vi "06. Native MQTT Instrument.vi"(11 "QualifiedName":string="demo/system/instrument") -> ()   [LabVIEW 2019]
uses:
  Actor/Request -- cluster.ctl
  <vilib>/LabVIEW Open Source Project/MQTT Control Packets/Control Packets/ControlPacket/ControlPacket.lvclass/ControlPacket.ctl
  eb005712-7d9b-4db0-ad4b-d7048dbf5e76.vi
  d83398bf-d288-4447-9c56-1851baa950d7.vi
  3288b219-43a6-48ac-a265-cf9a9541cd0b.vi
  5f2e3dba-ef2d-4927-820c-bacd114549c6.vi
  <vilib>/JDP Science/JSONtext/Find Item.vi
  <vilib>/JDP Science/JSONtext/Next JSON Value.vi
  <vilib>/JDP Science/JSONtext/String Subset.vi
  <vilib>/JDP Science/JSONtext/Parsing/Advance past next JSON Value (inlined COPY).vi
  <vilib>/JDP Science/JSONtext/Parsing/Advance past whitespace.vi
  <vilib>/JDP Science/JSONtext/Parsing/Advance past String.vi
  <vilib>/JDP Science/JSONtext/Parsing/Advance past Number.vi
  <vilib>/JDP Science/JSONtext/Parsing/Advance past Line Ending.vi
  <vilib>/LabVIEW Open Source Project/MQTT Control Packets/Control Packets/PUBLISH/PUBLISH.lvclass
  C:/Program Files (x86)/National Instruments/LabVIEW 2019/vi.lib/LabVIEW Open Source Project/MQTT Control Packets/Control Packets/ControlPacket/ControlPacket.lvclass
  <vilib>/JDP Science/JSONtext/JSON text to Variant.vi
  <vilib>/Utility/error.llb/Error Cluster From Error Code.vi
  <vilib>/JDP Science/JSONtext/Parsing/Parse Full Path or Item Name.vi
  <vilib>/JDP Science/JSONtext/Parsing/Advance past Array.vi
  <vilib>/JDP Science/JSONtext/Parsing/Advance past Object.vi
  <vilib>/JDP Science/JSONtext/support/Error Cluster From Code.vi
  <vilib>/JDP Science/JSONtext/Offset/Find Item Locations by Path.vi
  <vilib>/JDP Science/JSONtext/LVClass Serializer/JSONtext LVClass Serializer.lvclass
  <vilib>/ErrorRing/Error Ring.xnode
  <vilib>/LabVIEW Open Source Project/MQTT Control Packets/Control Packets/ControlPacket/ControlPacket.lvclass
  <vilib>/JDP Science/JSONtext/JSONtext.lvlib
  <vilib>/ptbypt/NI_PtbyPt.lvlib
panel:
  in  "amplitude":dbl
  out "<JSON>Response":string
  out "<JSON>":string caption="<JSON>Request"
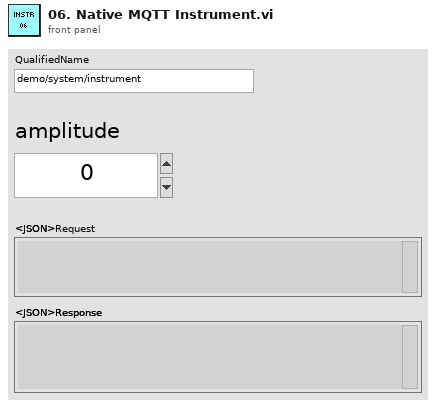
[diagram p1: front panel]
types:
  T1 = typedef "Actor Private Data.ctl" = cluster{"Client":refnum<class "Client.lvclass">, "QualifiedName":string, "EventReg":refnum<event-registration>, "Private Events":T2}
  T2 = typedef "Actor Private Events -- cluster.ctl" = cluster{"Stop":refnum<user-event>, "Subscribe":refnum<user-event>, "Unsubscribe":refnum<user-event>, "publish":refnum<user-event>}
  T3 = typedef "Request -- cluster.ctl" = cluster{"method":string, "<JSON>params":string, "id":string, "reply-topic":string}
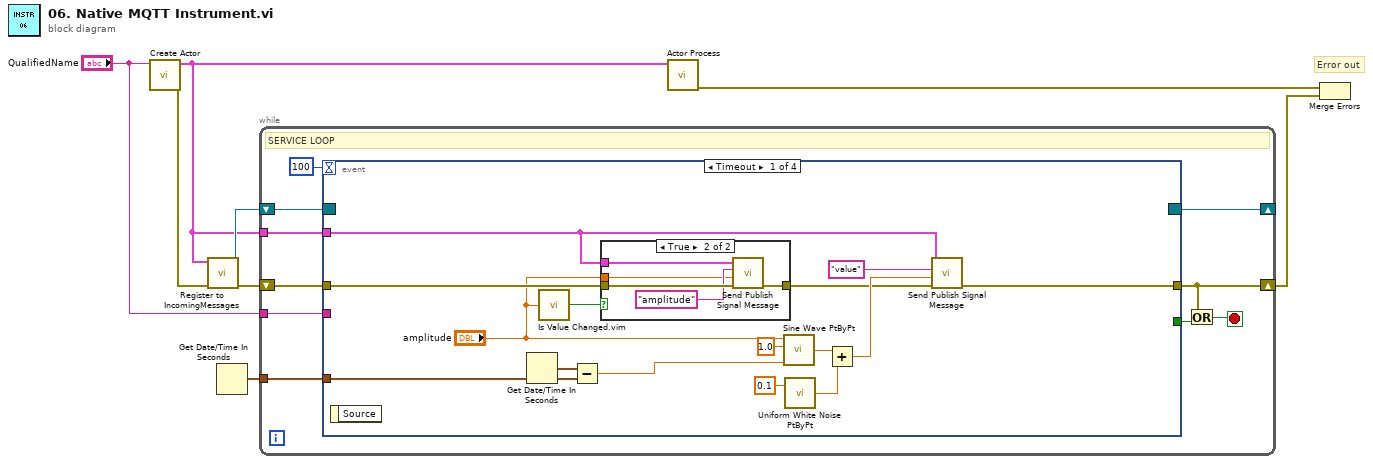
[diagram p0: block diagram]
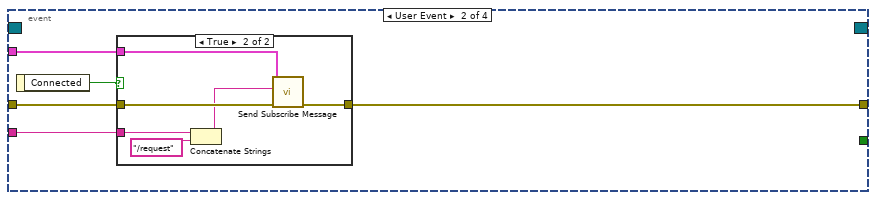
[diagram p3: hidden frame]
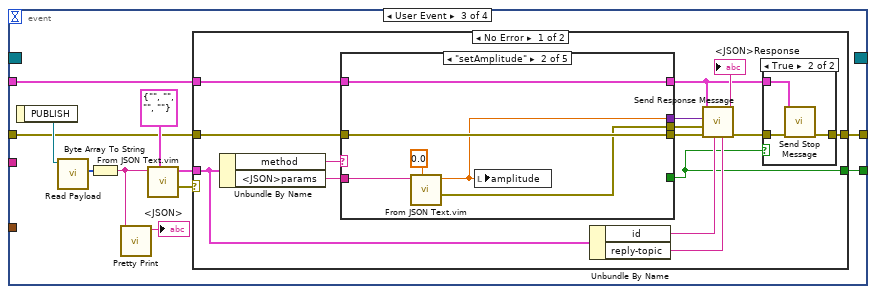
[diagram p5: hidden frame]
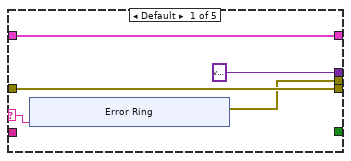
[diagram p7: hidden frame]
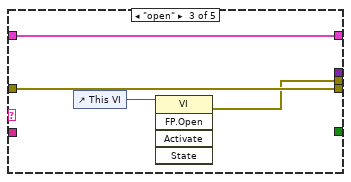
[diagram p8: hidden frame]
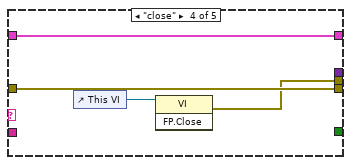
[diagram p9: hidden frame]
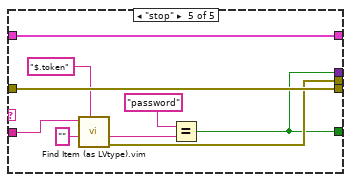
[diagram p10: hidden frame]
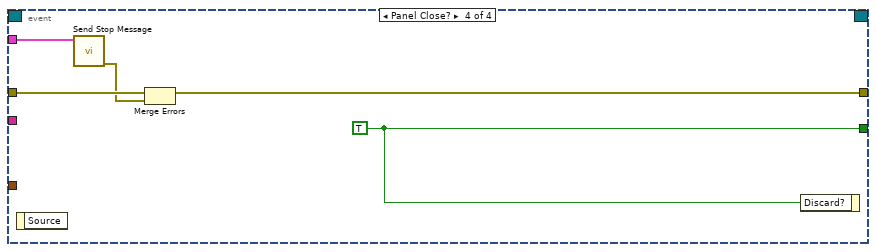
[diagram p12: hidden frame]
diagram:
  # "Error out"
  n1 = call "Create Actor.vi"("QualifiedName"="QualifiedName") -> ("error out"=w7:errorcluster, "Actor Class"=w5:T1)  [unwired: 9 in]
  n2 = call "Register to IncomingMessages.vi"("error in"=w7, "Actor Class"=w5) -> ("error out"=w4:errorcluster, "Incoming Messages"=w6:refnum<event-registration>)  [unwired: 8 in]
  n3 = Get Date/Time In Seconds() -> (seconds since 1Jan1904=w1:timestamp)
  n4 = while {
    tunnel: w5 -> [w16]
    shift-right: [w13] -> _
    shift-left: w6 -> [w14]
    shift-right: [w11] -> w3
    shift-left: w4 -> [w12]
    tunnel: "QualifiedName" -> [w10]
    tunnel: w1 -> [w9]
    stop <- w17 stop-if-true
    # "SERVICE LOOP"
    n5 = event shown="[0] Timeout" {
      selector: w14 -> [_ _ _ _]
      dyn-events: [_ _ _ _] -> w13
      timeout: 100 -> [_ _ _ _]
      tunnel: [_ _ w52 w122] -> w18
      tunnel: w16 -> [w24 w42 w57 w121]
      tunnel: [w28 w43 w55 w118] -> w11
      tunnel: w12 -> [w26 w44 w56 w120]
      tunnel: w10 -> [_ w40 _ _]
      tunnel: w9 -> [w20 _ _ _]
      event Timeout {
        n6 = event-data() -> ()  [unwired: 1 in, 1 out]
        n7 = Get Date/Time In Seconds() -> (seconds since 1Jan1904=w21:timestamp)
        n8 = call "Is Value Changed.vim"("value"="amplitude") -> ("changed or first call?"=w23:bool)
        n9 = Subtract(x=w21, y=w20) -> (x-y=w19:dbl)
        n10 = case shown="True" w23 {
          tunnel: w26 -> [w34 w39]
          tunnel: [w34 w38] -> w25
          tunnel: w24 -> [_ w36]
          tunnel: "amplitude" -> [_ w35]
          frame False {
          }
          frame True {
            n11 = call "Send Publish Signal Message.vi"("error in"=w39, "Variant"=w35, "Signal Name"="amplitude" ("Topic Name (empty: Payload name)"), "Actor Class"=w36) -> ("error out"=w38:errorcluster)  [unwired: 7 in]
          }
        }
        n12 = call <vilib>:"Sine Wave PtByPt.vi"("time"=w19, "frequency"=1.0, "amplitude"="amplitude") -> ("sine wave"=w33:dbl)  [unwired: 1 in]
        n13 = call <vilib>:"Uniform White Noise PtByPt.vi"("amplitude"=0.1) -> ("uniform white noise"=w31:dbl)  [unwired: 2 in]
        n14 = Add(x=w33, y=w31) -> (x+y=w29:dbl)
        n15 = call "Send Publish Signal Message.vi"("error in"=w25, "Variant"=w29, "Signal Name"="value" ("Topic Name (empty: Payload name)"), "Actor Class"=w24) -> ("error out"=w28:errorcluster)  [unwired: 7 in]
      }
      event User Event {
        n16 = event-data() -> ("Connected"=w41:bool)  [unwired: 1 in]
        n17 = case shown="True" w41 {
          tunnel: w44 -> [w45 w51]
          tunnel: [w45 w50] -> w43
          tunnel: w42 -> [_ w49]
          tunnel: w40 -> [_ w48]
          frame False {
          }
          frame True {
            n18 = Concatenate Strings(w48, "/request" ("QualifiedName")) -> (w46:string)
            n19 = call "Send Subscribe Message.vi"("error in"=w51, "Topic"=w46, "Actor Class"=w49) -> ("error out"=w50:errorcluster)  [unwired: 8 in]
          }
        }
      }
      event User Event {
        n20 = event-data() -> ("PUBLISH"=w62:refnum<class "PUBLISH.lvclass">)  [unwired: 1 in]
        n21 = call <vilib>:"Read Payload.vi"("ControlPacket in"=w62) -> ("Payload"=w61:u8[])  [unwired: 9 in, 1 out]
        n22 = Byte Array To String(unsigned byte array=w61) -> (string=w54:string)
        n23 = call <vilib>:"Pretty Print.vi"("JSON"=w54) -> ("<JSON>"=→"<JSON>":string)  [unwired: 8 in, 2 out]
        n24 = call "From JSON Text.vim"("Data Type and Default Value"=T3 {"method"="", "<JSON>params"="", "id"="", "reply-topic"=""} ("request"), "JSON"=w54) -> ("error out"=w59:errorcluster, "Data out"=w58:T3)  [unwired: 8 in]
        n25 = case shown="No Error" w59 {
          tunnel: w58 -> [w68 _]
          tunnel: w57 -> [w75 _]
          tunnel: w56 -> [w74 w117]
          tunnel: [w65 w117] -> w55
          tunnel: [w63 _] -> w52
          frame No Error {
            n26 = Unbundle By Name(w68) -> ("method"=w77:string, "<JSON>params"=w76:string)
            n27 = case shown="\"setAmplitude\"" w77 {
              selector: w77 -> [w82 _ _ _ _]
              tunnel: w76 -> [_ w97 _ _ w114]
              tunnel: w75 -> [w85 w98 w103 w107 w115]
              tunnel: w74 -> [w86 w99 w101 w105 w116]
              tunnel: [w86 w99 w101 w105 w116] -> w73
              tunnel: [w85 w98 w103 w107 w115] -> w64
              tunnel: [w84 w94 w100 w104 w109] -> w70
              tunnel: [variant ("result") w95 _ _ w108] -> w69
              tunnel: [_ _ _ _ w108] -> w63
              frame Default {
                n28 = xnode "Error Ring"("parameter 0"=w82) -> ("error out"=w84:errorcluster)
              }
              frame "setAmplitude" {
                n29 = call "From JSON Text.vim"("Data Type and Default Value"=0.0, "JSON"=w97) -> ("error out"=w94:errorcluster, "Data out"=w95:dbl)  [unwired: 8 in]
                n30 = local write "amplitude"(w95) -> ()
              }
              frame "open" {
                n31 = control-ref of="This VI"() -> (w102:refnum<vi>)
                n32 = invoke class="VI" method="FP.Open"(reference=w102) -> (error out=w100:errorcluster)  [unwired: 4 in, 4 out]
              }
              frame "close" {
                n33 = control-ref of="This VI"() -> (w106:refnum<vi>)
                n34 = invoke class="VI" method="FP.Close"(reference=w106) -> (error out=w104:errorcluster)  [unwired: 2 in, 2 out]
              }
              frame "stop" {
                n35 = call "Find Item (as LVtype).vim"("$Path or Item Name"="$.token", "Data Type and Default Value"="", "JSON"=w114) -> ("error out"=w109:errorcluster, "Data"=w111:string)  [unwired: 5 in, 2 out]
                n36 = Equal?(x="password" ("$Path or Item Name"), y=w111) -> (x = y?=w108:bool)
              }
            }
            n37 = Unbundle By Name(w68) -> ("id"=w72:string, "reply-topic"=w71:string)
            n38 = call "Send Response Message.vi"("topic"=w71, "id"=w72, "error in"=w73, "request error"=w70, "result"=w69, "Actor Class"=w64) -> ("error out"=w66:errorcluster, "<JSON>Response"=→"<JSON>Response":string)  [unwired: 4 in]
            n39 = case shown="True" w63 {
              tunnel: w66 -> [w78 w81]
              tunnel: [w78 w80] -> w65
              tunnel: w64 -> [_ w79]
              frame False {
              }
              frame True {
                n40 = call "Send Stop Message.vi"("error in"=w81, "Actor Class"=w79) -> ("error out"=w80:errorcluster)  [unwired: 9 in]
              }
            }
          }
          frame Error {
            # "Invalid request payload"
          }
        }
      }
      event Panel Close? {
        w122 = TRUE ("Discard?")
        n41 = event-data() -> ()  [unwired: 1 in, 1 out]
        n42 = call "Send Stop Message.vi"("Actor Class"=w121) -> ("error out"=w119:errorcluster)  [unwired: 10 in]
        n43 = Merge Errors(w120, w119) -> (w118:errorcluster)
        n44 = event-data("Discard?"=w122) -> ()  [unwired: 1 in, 1 out]
      }
    }
    n45 = Or(x=w11, y=w18) -> (x .or. y?=w17:bool)
  }
  n46 = call "Actor Process.vi"("Actor Class"=w5) -> ("error out"=w8:errorcluster)  [unwired: 10 in]
  n47 = Merge Errors(w8, w3) -> ()  [unwired: 1 out]
